vi "Inverse DCT.vi"   [LabVIEW 2020, in "NI_AALPro.lvlib"]
doc: "Computes the inverse Discrete Cosine Transform (DCT) of the input sequence <B>DCT {X}</B>. Wire data to the <B>DCT {X}</B> input to determine the polymorphic instance to use or manually select the instance."
uses:
  NI_AALPro.lvlib
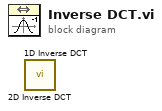
[diagram p0: block diagram]
diagram:
  n1 = call "2D Inverse DCT.vi"() -> ()  [unwired: 10 in, 2 out]
  n2 = call "1D Inverse DCT.vi"() -> ()  [unwired: 10 in, 2 out]
